vi "lvsocket write.vi"(8 "error in":errorcluster, 10 "data":string, 11 "tls context":u64) -> (0 "error out":errorcluster, 3 "error response":i32)   [LabVIEW 2016, in "lv tls dll.lvlib"]
uses:
  lv tls dll.lvlib
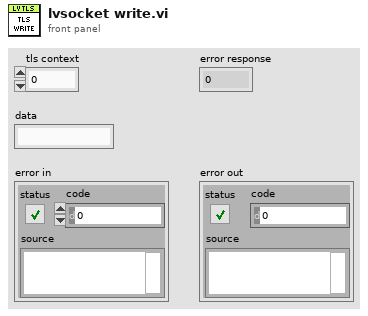
[diagram p1: front panel]
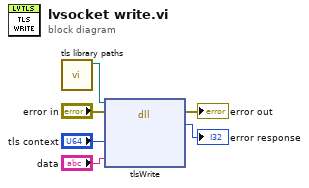
[diagram p0: block diagram]
diagram:
  n1 = call "tls library paths.vi"() -> ("lvtls"=w1:path)  [unwired: 8 in, 3 out]
  n2 = dll-call lib="C:/Users/IEUser/Desktop/tlssimple/lvlibtls.dll" fn="tlsWrite"(path in=w1, error in="error in", "context"="tls context", "data"="data") -> (error out=→"error out":errorcluster, "err"=→"error response":i32)  [unwired: 3 in, 1 out]
